vi "midi out close.vi"(7 "MIDI output handle":i32) -> (0 "Win32 error code":i32)   [LabVIEW 2016]
doc: "Closes a reference to a MIDI output device."
uses:
  winmm.dll
panel:
  # "Select Help»Show Context Help and move the cursor over the VI icon to display help for this VI."
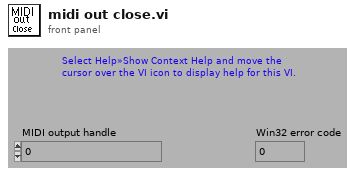
[diagram p1: front panel]
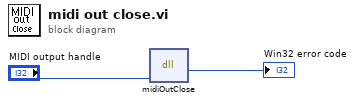
[diagram p0: block diagram]
diagram:
  n1 = dll-call lib="winmm.dll" fn="midiOutClose"("hmidiout"="MIDI output handle") -> (→"Win32 error code":i32)  [unwired: 4 in, 2 out]
